vi "Write Time Info.vi"(0 "Request Data in":refnum<class "Timed Data.lvclass">, 5 "Start TIme":timestamp, 7 "Duration(s)":dbl, 9 "Data ID":u32, 11 "error in (no error)":errorcluster) -> (4 "Request Data out":refnum<class "Timed Data.lvclass">, 15 "error out":errorcluster)   [LabVIEW 2020, in "Publisher.lvlib" / "Timed Data.lvclass"]
doc: "Write Start Time, Duration and DataID to the Timed Data."
uses:
  Timed Data.lvclass
  Timed Data.lvclass/Timed Data.ctl
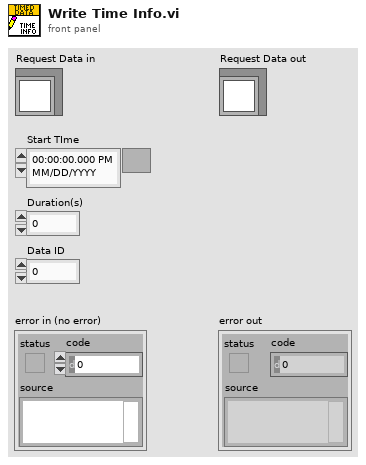
[diagram p1: front panel]
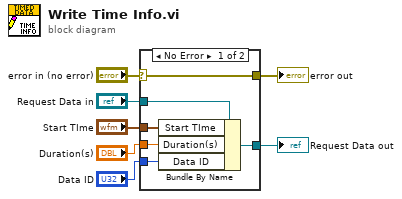
[diagram p0: block diagram]
diagram:
  n1 = case shown="No Error" "error in (no error)" {
    selector: "error in (no error)" -> [w13 w14]
    tunnel: [w13 w14] -> w6
    tunnel: [w11 w15] -> w4
    tunnel: "Request Data in" -> [w12 w15]
    tunnel: "Start TIme" -> [w10 _]
    tunnel: "Duration(s)" -> [w9 _]
    tunnel: "Data ID" -> [w8 _]
    frame No Error {
      n2 = Bundle By Name(cluster=w12, "Start TIme"=w10, "Duration(s)"=w9, "Data ID"=w8) -> (w11:refnum<class "Timed Data.lvclass">)
    }
    frame Error {
    }
  }
  "error out" <- w6
  "Request Data out" <- w4
